vi "Create Broadcast Enqueuer References.vi"(8 "error in (no error)":errorcluster) -> (0 "error out":errorcluster, 3 "Broadcasts":T1)   [LabVIEW 2018, in "Scripting.lvlib" / "Actor.lvclass"]
uses:
  Actor.lvclass
  Broadcast Enqueuers.ctl
  Did Initialize.ctl
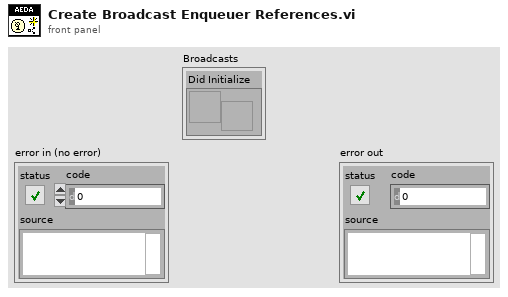
[diagram p1: front panel]
types:
  T1 = typedef "Scripting.lvlib/Actor.lvclass/Broadcast Enqueuers.ctl" = cluster{"Did Initialize":refnum<user-event>}
  T2 = typedef "Scripting.lvlib/Actor.lvclass/Did Initialize.ctl" = cluster{"State":refnum<class "Actor.lvclass">}
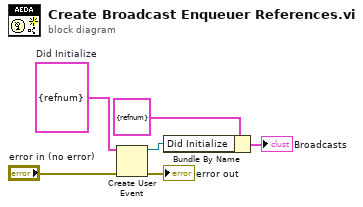
[diagram p0: block diagram]
diagram:
  w3 = T2 {"State"=refnum}  # Did Initialize
  n1 = Create User Event(user event datatype=w3, error in="error in (no error)") -> (user event=w2:refnum<user-event>, error out=→"error out":errorcluster)
  n2 = Bundle By Name(cluster=T1 {"Did Initialize"=refnum} ("Broadcast Enqueuers"), "Did Initialize"=w2) -> (→"Broadcasts":T1)
